vi "set log location.vi"(8 "error in (no error)":errorcluster, 11 "log directory":path) -> (0 "error out":errorcluster)   [LabVIEW 2024, in "atsj peakcan basic.lvlib"]
uses:
  atsj peakcan basic.lvlib
  parameter.ctl
  set parameter - string.vi
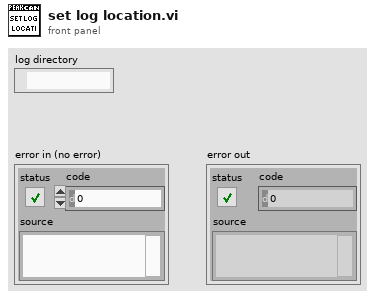
[diagram p1: front panel]
types:
  T1 = typedef "atsj peakcan basic.lvlib/parameter.ctl" = enum8{"DEVICE_ID", "5VOLTS_POWER", "RECEIVE_EVENT", "MESSAGE_FILTER", "API_VERSION", "CHANNEL_VERSION", "BUSOFF_AUTORESET", "LISTEN_ONLY", "LOG_LOCATION", "LOG_STATUS", "LOG_CONFIGURE", "LOG_TEXT", "CHANNEL_CONDITION", "HARDWARE_NAME", "RECEIVE_STATUS", "CONTROLLER_NUMBER", "TRACE_LOCATION", "TRACE_STATUS", "TRACE_SIZE", "TRACE_CONFIGURE", "CHANNEL_IDENTIFYING", "CHANNEL_FEATURES", "BITRATE_ADAPTING", "BITRATE_INFO", "BITRATE_INFO_FD", "BUSSPEED_NOMINAL", "BUSSPEED_DATA", "IP_ADDRESS", "LAN_SERVICE_STATUS", "ALLOW_STATUS_FRAMES", "ALLOW_RTR_FRAMES", "ALLOW_ERROR_FRAMES", "INTERFRAME_DELAY", "ACCEPTANCE_FILTER_11BIT", "ACCEPTANCE_FILTER_29BIT", "IO_DIGITAL_CONFIGURATION", "IO_DIGITAL_VALUE", "IO_DIGITAL_SET", "IO_DIGITAL_CLEAR", "IO_ANALOG_VALUE", "FIRMWARE_VERSION", "ATTACHED_CHANNELS_COUNT", "ATTACHED_CHANNELS", "ALLOW_ECHO_FRAMES", "DEVICE_PART_NUMBER", "HARD_RESET_STATUS", "LAN_CHANNEL_DIRECTION", "DEVICE_GUID"}
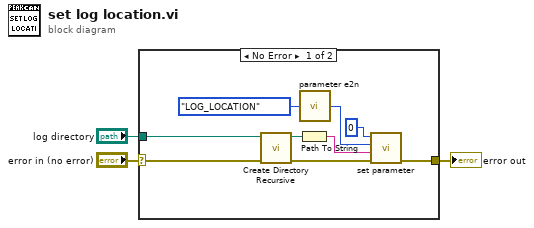
[diagram p0: block diagram]
diagram:
  n1 = case shown="No Error" "error in (no error)" {
    selector: "error in (no error)" -> [w6 w13]
    tunnel: [w5 w13] -> w2
    tunnel: "log directory" -> [w4 _]
    frame No Error {
      n2 = call <vilib>:"Create Directory Recursive.vi"("error in (no error)"=w6, "directory"=w4) -> ("error out"=w9:errorcluster, "directory copy"=w10:path)  [unwired: 3 in, 1 out]
      n3 = Path To String(path=w10) -> (string=w11:string)
      n4 = call "parameter e2n.vi"("parameter"=parameter."LOG_LOCATION") -> ("number"=w7:u8)
      n5 = call-poly "set parameter.vi"("error in (no error)"=w9, "value"=w11, "parameter"=w7, "channel"=u16 0) -> ("error out"=w5:errorcluster)  [unwired: 7 in]
    }
    frame Error {
    }
  }
  "error out" <- w2
